vi "VIPB to VIPM variant.vi"(9 "LVProj":path, 10 "Path to VIPB File":path) -> (2 "Variant":variant)   [LabVIEW 2019, in "VIPM.lvlib"]
uses:
  VIPM.lvlib
panel:
  out "error out":errorcluster
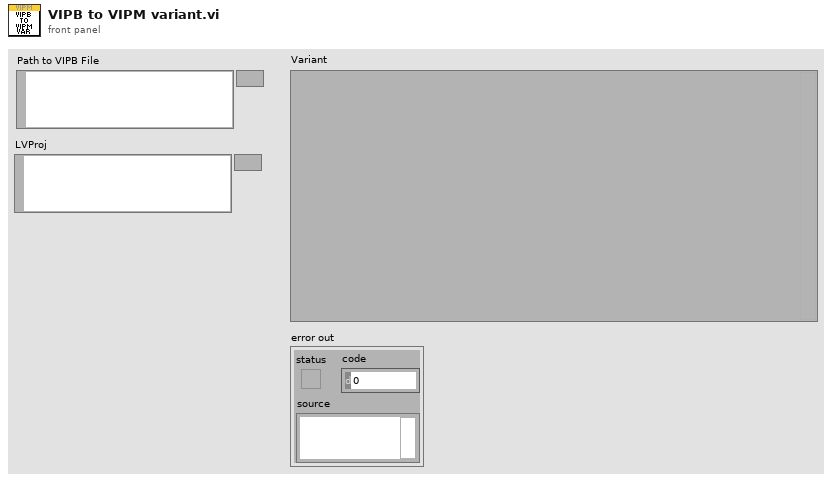
[diagram p1: front panel]
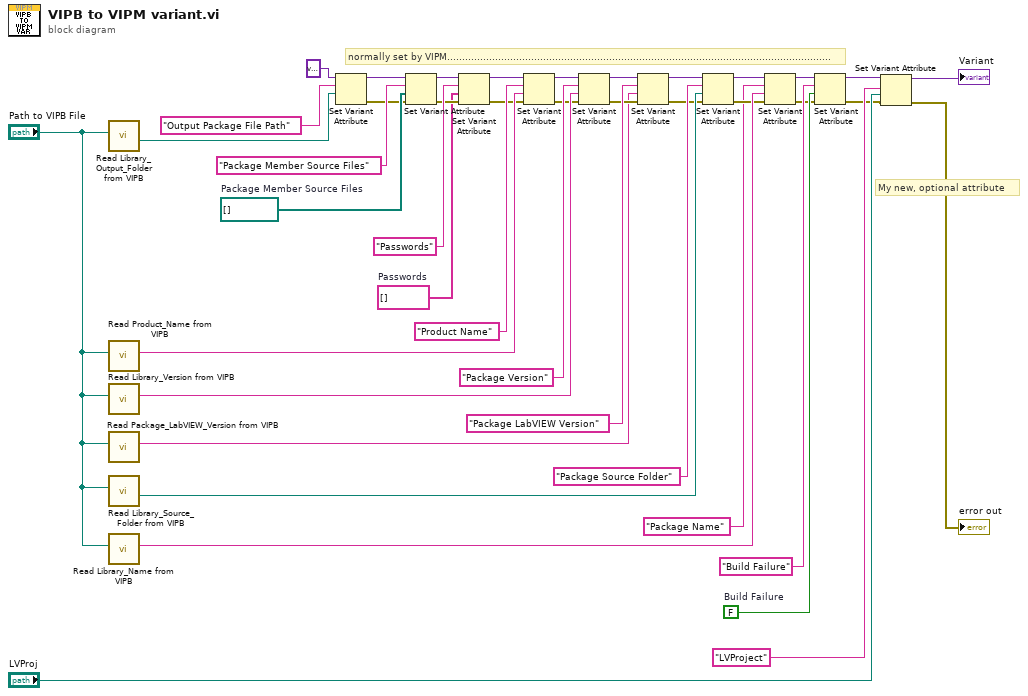
[diagram p0: block diagram]
diagram:
  w36 = FALSE  # Build Failure
  w8 = string[] []  # Passwords
  w42 = path[] []  # Package Member Source Files
  # "My new, optional attribute"
  # "normally set by VIPM................................................................................................................................"
  n1 = call "Read Library_Output_Folder from VIPB.vi"("VIPB File Path"="Path to VIPB File") -> ("appended path"=w11:path)  [unwired: 8 in, 2 out]
  n2 = call "Read Product_Name from VIPB.vi"("VIPB File Path"="Path to VIPB File") -> ("Product_Name"=w23:string)  [unwired: 9 in, 1 out]
  n3 = call "Read Library_Version from VIPB.vi"("VIPB File Path"="Path to VIPB File") -> ("Library_Version"=w24:string)  [unwired: 9 in, 1 out]
  n4 = call "Read Package_LabVIEW_Version from VIPB.vi"("VIPB File Path"="Path to VIPB File") -> ("Package_LabVIEW_Version"=w9:string)  [unwired: 9 in, 1 out]
  n5 = call "Read Library_Source_Folder from VIPB.vi"("VIPB File Path"="Path to VIPB File") -> ("appended path"=w25:path)  [unwired: 8 in, 2 out]
  n6 = call "Read Library_Name from VIPB.vi"("VIPB File Path"="Path to VIPB File") -> ("Package_Name"=w22:string)  [unwired: 9 in, 1 out]
  n7 = Set Variant Attribute(Variant=variant ("variant"), name="Output Package File Path", value=w11) -> (Variant out=w27:variant, error out=w20:errorcluster)  [unwired: 1 in, 1 out]
  n8 = Set Variant Attribute(Variant=w27, name="Package Member Source Files", value=w42, error in=w20) -> (Variant out=w28:variant, error out=w19:errorcluster)  [unwired: 1 out]
  n9 = Set Variant Attribute(Variant=w28, name="Passwords", value=w8, error in=w19) -> (Variant out=w29:variant, error out=w18:errorcluster)  [unwired: 1 out]
  n10 = Set Variant Attribute(Variant=w29, name="Product Name", value=w23, error in=w18) -> (Variant out=w30:variant, error out=w17:errorcluster)  [unwired: 1 out]
  n11 = Set Variant Attribute(Variant=w30, name="Package Version", value=w24, error in=w17) -> (Variant out=w31:variant, error out=w16:errorcluster)  [unwired: 1 out]
  n12 = Set Variant Attribute(Variant=w31, name="Package LabVIEW Version", value=w9, error in=w16) -> (Variant out=w32:variant, error out=w15:errorcluster)  [unwired: 1 out]
  n13 = Set Variant Attribute(Variant=w32, name="Package Source Folder", value=w25, error in=w15) -> (Variant out=w33:variant, error out=w14:errorcluster)  [unwired: 1 out]
  n14 = Set Variant Attribute(Variant=w33, name="Package Name", value=w22, error in=w14) -> (Variant out=w34:variant, error out=w12:errorcluster)  [unwired: 1 out]
  n15 = Set Variant Attribute(Variant=w34, name="Build Failure", value=w36, error in=w12) -> (Variant out=w6:variant, error out=w2:errorcluster)  [unwired: 1 out]
  n16 = Set Variant Attribute(Variant=w6, name="LVProject", value="LVProj", error in=w2) -> (Variant out=→"Variant":variant, error out=→"error out":errorcluster)  [unwired: 1 out]
